vi "EnumDevicesEx.vi"(5 "nLayerType":u32=1, 11 "error in (no error)":errorcluster caption="错误输入（无错误）") -> (4 "function return":i32, 6 "nDeviceNumReturn":u32, 8 "GigEDeviceArray":T2(array[cluster]), 10 "U3VDeviceArray":T1(array[cluster]), 15 "error out":errorcluster caption="错误输出")   [LabVIEW 2013, in "MvCameraControl.lvlib"]
uses:
  MvCameraControl.lvlib
  MvCameraPatch.dll
panel:
  in  "strManufacturerName":i8[](array[numeric])
  in  "U3VDevice":T3
  in  "GigEDevice":T4
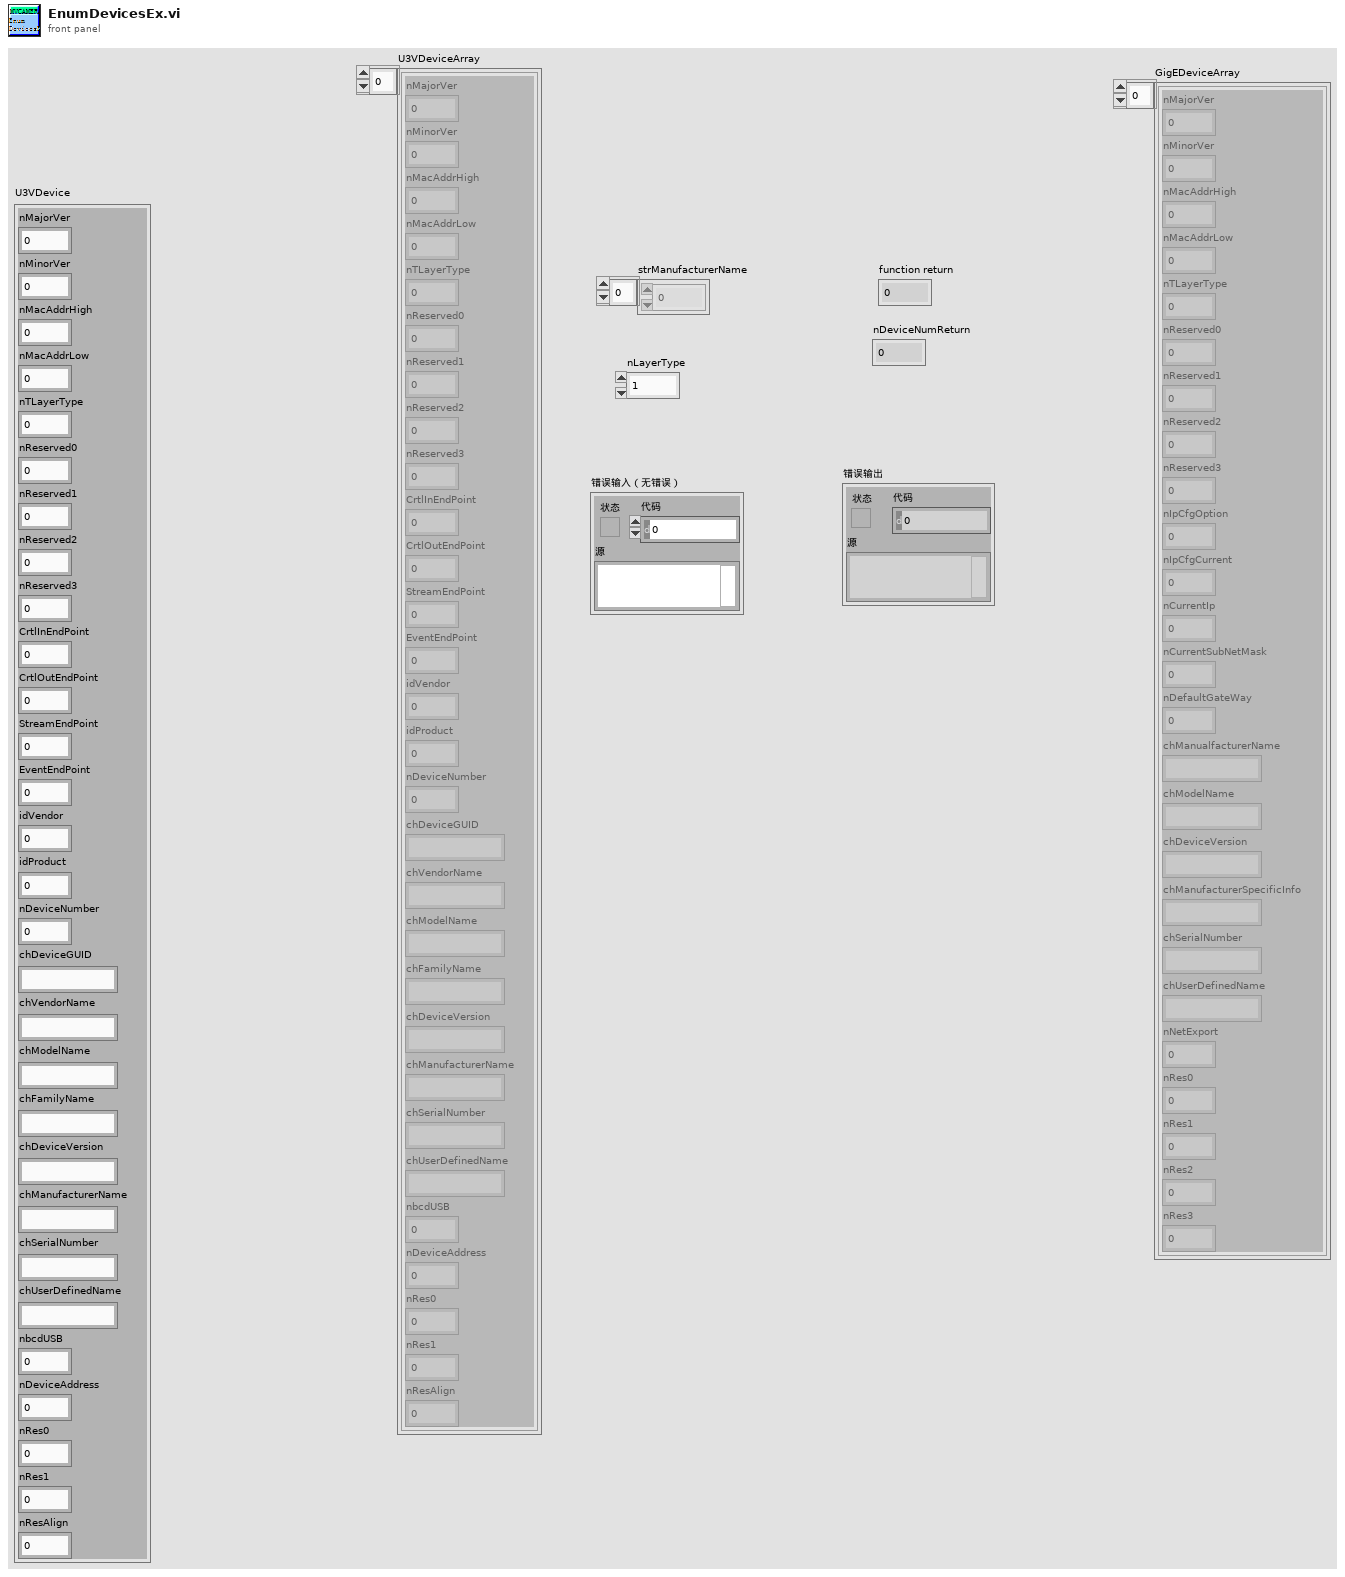
[diagram p1: front panel]
types:
  T1 = cluster{"nMajorVer":u16, "nMinorVer":u16, "nMacAddrHigh":u32, "nMacAddrLow":u32, "nTLayerType":u32, "nReserved0":u32, "nReserved1":u32, "nReserved2":u32, "nReserved3":u32, "CrtlInEndPoint":u8, "CrtlOutEndPoint":u8, "StreamEndPoint":u8, "EventEndPoint":u8, "idVendor":u16, "idProduct":u16, "nDeviceNumber":u32, "chDeviceGUID":string, "chVendorName":string, "chModelName":string, "chFamilyName":string, "chDeviceVersion":string, "chManufacturerName":string, "chSerialNumber":string, "chUserDefinedName":string, "nbcdUSB":u32, "nDeviceAddress":u32, "nRes0":u32, "nRes1":u32, "nResAlign":u32}[]
  T2 = cluster{"nMajorVer":u16, "nMinorVer":u16, "nMacAddrHigh":u32, "nMacAddrLow":u32, "nTLayerType":u32, "nReserved0":u32, "nReserved1":u32, "nReserved2":u32, "nReserved3":u32, "nIpCfgOption":u32, "nIpCfgCurrent":u32, "nCurrentIp":u32, "nCurrentSubNetMask":u32, "nDefaultGateWay":u32, "chManualfacturerName":string, "chModelName":string, "chDeviceVersion":string, "chManufacturerSpecificInfo":string, "chSerialNumber":string, "chUserDefinedName":string, "nNetExport":u32, "nRes0":u32, "nRes1":u32, "nRes2":u32, "nRes3":u32}[]
  T3 = cluster{"nMajorVer":u16, "nMinorVer":u16, "nMacAddrHigh":u32, "nMacAddrLow":u32, "nTLayerType":u32, "nReserved0":u32, "nReserved1":u32, "nReserved2":u32, "nReserved3":u32, "CrtlInEndPoint":u8, "CrtlOutEndPoint":u8, "StreamEndPoint":u8, "EventEndPoint":u8, "idVendor":u16, "idProduct":u16, "nDeviceNumber":u32, "chDeviceGUID":string, "chVendorName":string, "chModelName":string, "chFamilyName":string, "chDeviceVersion":string, "chManufacturerName":string, "chSerialNumber":string, "chUserDefinedName":string, "nbcdUSB":u32, "nDeviceAddress":u32, "nRes0":u32, "nRes1":u32, "nResAlign":u32}
  T4 = cluster{"nMajorVer":u16, "nMinorVer":u16, "nMacAddrHigh":u32, "nMacAddrLow":u32, "nTLayerType":u32, "nReserved0":u32, "nReserved1":u32, "nReserved2":u32, "nReserved3":u32, "nIpCfgOption":u32, "nIpCfgCurrent":u32, "nCurrentIp":u32, "nCurrentSubNetMask":u32, "nDefaultGateWay":u32, "chManualfacturerName":string, "chModelName":string, "chDeviceVersion":string, "chManufacturerSpecificInfo":string, "chSerialNumber":string, "chUserDefinedName":string, "nNetExport":u32, "nRes0":u32, "nRes1":u32, "nRes2":u32, "nRes3":u32}
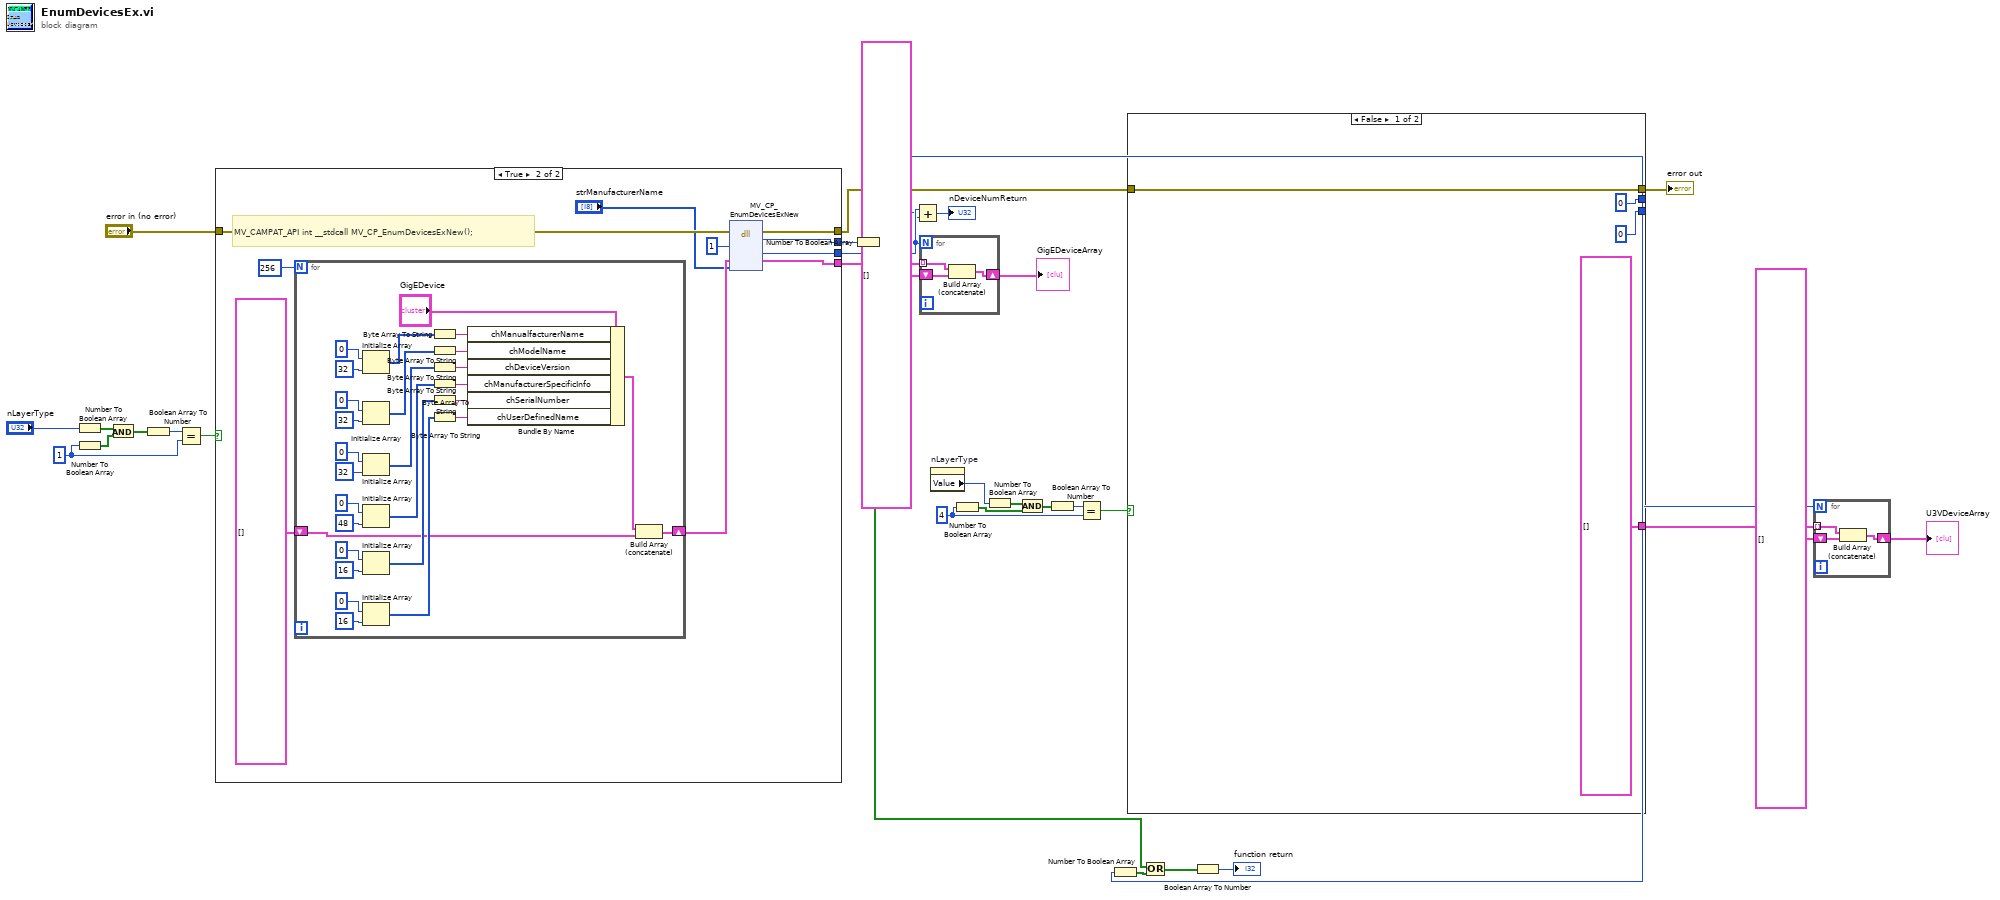
[diagram p0: block diagram]
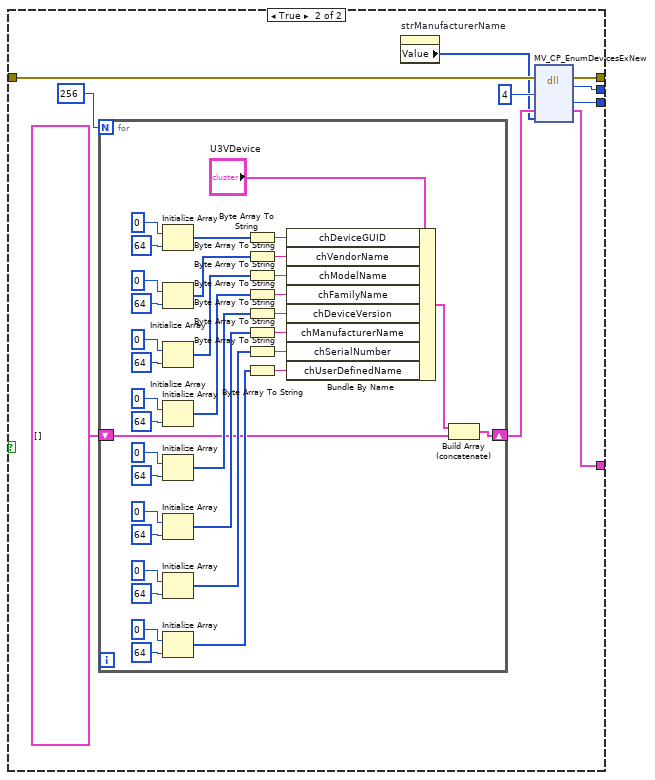
[diagram p2: hidden frame]
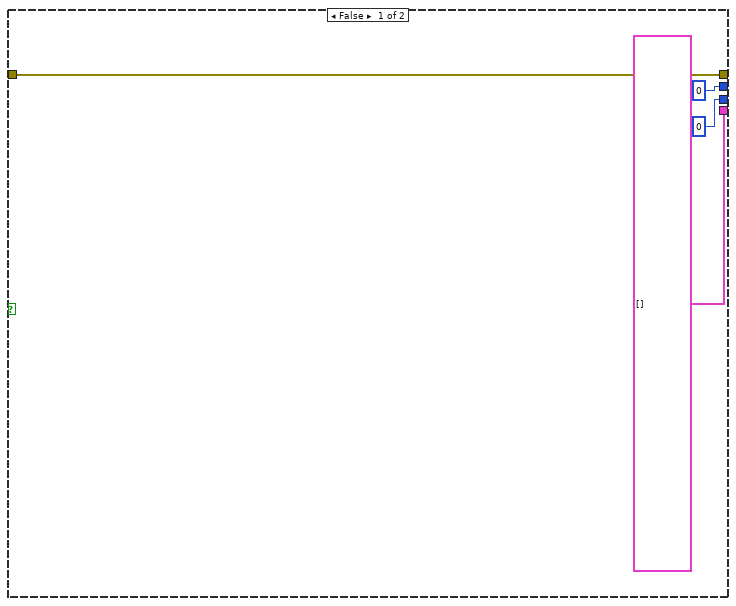
[diagram p3: hidden frame]
diagram:
  w20 = u32 4 ("数字")
  w28 = u32 1 ("数字")
  n1 = Number To Boolean Array(number="nLayerType") -> (Boolean array=w32:bool[])
  n2 = Number To Boolean Array(number=w28) -> (Boolean array=w31:bool[])
  n3 = And(x=w32, y=w31) -> (x .and. y?=w30:bool[])
  n4 = Boolean Array To Number(Boolean array=w30) -> (number=w29:u32)
  n5 = Equal?(x=w29, y=w28) -> (x = y?=w27:bool)
  n6 = case shown="True" w27 {
    tunnel: [0 ("返回类型") w43] -> w16
    tunnel: [u32 0 ("nDeviceNumReturn") w42] -> w9
    tunnel: "error in (no error)" -> [w34 w41]
    tunnel: [w34 w40] -> w11
    tunnel: [T2 [] ("DeviceInfoArray") w38] -> w6
    frame False {
    }
    frame True {
      # "MV_CAMPAT_API int __stdcall MV_CP_EnumDevicesExNew();"
      n7 = for {
        N: 256 -> [_]
        shift-right: [w49] -> w46
        shift-left: T2 [] -> [w47]
        n8 = Initialize Array(u8 0 ("元素"), 32 ("维数大小")) -> (w58:u8[])
        n9 = Initialize Array(u8 0 ("元素"), 32 ("维数大小")) -> (w61:u8[])
        n10 = Initialize Array(u8 0 ("元素"), 32 ("维数大小")) -> (w50:u8[])
        n11 = Initialize Array(u8 0 ("元素"), 48 ("维数大小")) -> (w55:u8[])
        n12 = Initialize Array(u8 0 ("元素"), 16 ("维数大小")) -> (w69:u8[])
        n13 = Initialize Array(u8 0 ("元素"), 16 ("维数大小")) -> (w66:u8[])
        n14 = Byte Array To String(unsigned byte array=w58) -> (string=w70:string)
        n15 = Byte Array To String(unsigned byte array=w61) -> (string=w71:string)
        n16 = Byte Array To String(unsigned byte array=w50) -> (string=w51:string)
        n17 = Byte Array To String(unsigned byte array=w55) -> (string=w72:string)
        n18 = Byte Array To String(unsigned byte array=w69) -> (string=w73:string)
        n19 = Byte Array To String(unsigned byte array=w66) -> (string=w74:string)
        n20 = Bundle By Name(cluster="GigEDevice", "chManualfacturerName"=w70, "chModelName"=w71, "chDeviceVersion"=w51, "chManufacturerSpecificInfo"=w72, "chSerialNumber"=w73, "chUserDefinedName"=w74) -> (w48:T4)
        n21 = Build Array (concatenate)(w48, w47) -> (w49:T2)
      }
      n22 = dll-call lib="MvCameraPatch.dll" fn="MV_CP_EnumDevicesExNew"(error in=w41, "nLayerType"=u32 1, "DeviceInfoArray"=w46, "strManufacturerName"="strManufacturerName") -> (error out=w40:errorcluster, "返回类型"=w43:i32, "nDeviceNumReturn"=w42:u32, "DeviceInfoArray"=w38:T2)  [unwired: 5 in, 1 out]
    }
  }
  n23 = Number To Boolean Array(number=w16) -> (Boolean array=w15:bool[])
  n24 = for {
    N: w9 -> [_]
    tunnel: w6 -> [w77] mode=indexing
    shift-right: [w75] -> w4
    shift-left: T2 [] -> [w76]
    n25 = Build Array (concatenate)(w77, w76) -> (w75:T2)
  }
  "GigEDeviceArray" <- w4
  n26 = property on="nLayerType" class="DigNum (strict)"() -> ("Value"=w7:u32)  [unwired: 2 in, 2 out]
  n27 = Number To Boolean Array(number=w20) -> (Boolean array=w23:bool[])
  n28 = Number To Boolean Array(number=w7) -> (Boolean array=w24:bool[])
  n29 = And(x=w24, y=w23) -> (x .and. y?=w22:bool[])
  n30 = Boolean Array To Number(Boolean array=w22) -> (number=w21:u32)
  n31 = Equal?(x=w21, y=w20) -> (x = y?=w19:bool)
  n32 = case shown="False" w19 {
    tunnel: [u32 0 ("nDeviceNumReturn") w90] -> w8
    tunnel: [0 ("返回类型") w89] -> w17
    tunnel: w11 -> [w79 w88]
    tunnel: [w79 w87] -> w10
    tunnel: [T1 [] w83] -> w3
    frame False {
    }
    frame True {
      n33 = for {
        N: 256 -> [_]
        shift-right: [w92] -> w85
        shift-left: T1 [] -> [w94]
        n34 = Initialize Array(u8 0 ("元素"), 64 ("维数大小")) -> (w98:u8[])
        n35 = Initialize Array(u8 0 ("元素"), 64 ("维数大小")) -> (w102:u8[])
        n36 = Initialize Array(u8 0 ("元素"), 64 ("维数大小")) -> (w105:u8[])
        n37 = Initialize Array(u8 0 ("元素"), 64 ("维数大小")) -> (w108:u8[])
        n38 = Initialize Array(u8 0 ("元素"), 64 ("维数大小")) -> (w111:u8[])
        n39 = Initialize Array(u8 0 ("元素"), 64 ("维数大小")) -> (w114:u8[])
        n40 = Initialize Array(u8 0 ("元素"), 64 ("维数大小")) -> (w121:u8[])
        n41 = Initialize Array(u8 0 ("元素"), 64 ("维数大小")) -> (w126:u8[])
        n42 = Byte Array To String(unsigned byte array=w98) -> (string=w99:string)
        n43 = Byte Array To String(unsigned byte array=w102) -> (string=w115:string)
        n44 = Byte Array To String(unsigned byte array=w105) -> (string=w116:string)
        n45 = Byte Array To String(unsigned byte array=w108) -> (string=w117:string)
        n46 = Byte Array To String(unsigned byte array=w111) -> (string=w118:string)
        n47 = Byte Array To String(unsigned byte array=w114) -> (string=w122:string)
        n48 = Byte Array To String(unsigned byte array=w121) -> (string=w123:string)
        n49 = Byte Array To String(unsigned byte array=w126) -> (string=w127:string)
        n50 = Bundle By Name(cluster="U3VDevice", "chDeviceGUID"=w99, "chVendorName"=w115, "chModelName"=w116, "chFamilyName"=w117, "chDeviceVersion"=w118, "chManufacturerName"=w122, "chSerialNumber"=w123, "chUserDefinedName"=w127) -> (w93:T3)
        n51 = Build Array (concatenate)(w93, w94) -> (w92:T1)
      }
      n52 = property on="strManufacturerName" class="Arr (strict)"() -> ("Value"=w82:i8[])  [unwired: 2 in, 2 out]
      n53 = dll-call lib="MvCameraPatch.dll" fn="MV_CP_EnumDevicesExNew"(error in=w88, "nLayerType"=u32 4, "DeviceInfoArray"=w85, "strManufacturerName"=w82) -> (error out=w87:errorcluster, "返回类型"=w89:i32, "nDeviceNumReturn"=w90:u32, "DeviceInfoArray"=w83:T1)  [unwired: 5 in, 1 out]
    }
  }
  "error out" <- w10
  n54 = Add(x=w9, y=w8) -> (x+y=→"nDeviceNumReturn":u32)
  n55 = Number To Boolean Array(number=w17) -> (Boolean array=w14:bool[])
  n56 = Or(x=w15, y=w14) -> (x .or. y?=w13:bool[])
  n57 = Boolean Array To Number(Boolean array=w13) -> (number=→"function return":u32)
  n58 = for {
    N: w8 -> [_]
    tunnel: w3 -> [w130] mode=indexing
    shift-right: [w128] -> w1
    shift-left: T1 [] -> [w129]
    n59 = Build Array (concatenate)(w130, w129) -> (w128:T1)
  }
  "U3VDeviceArray" <- w1
